vi "Bundler_Move Up Down Element Order.vi"(7 "Action":T2=enum."Bundler Move Up", 10 "Cluster Elements In":T1[](array[typedef]), 11 "Affected Items":T3) -> (3 "Cluster Elements Out":T1[](array[typedef]))   [LabVIEW 2023]
uses:
  top/BundleMagic.ctl
  controls/action enum.ctl
  Cluster Element Description.ctl
panel:
  # "Using Bundler Move Up and Bundler Move Down only"
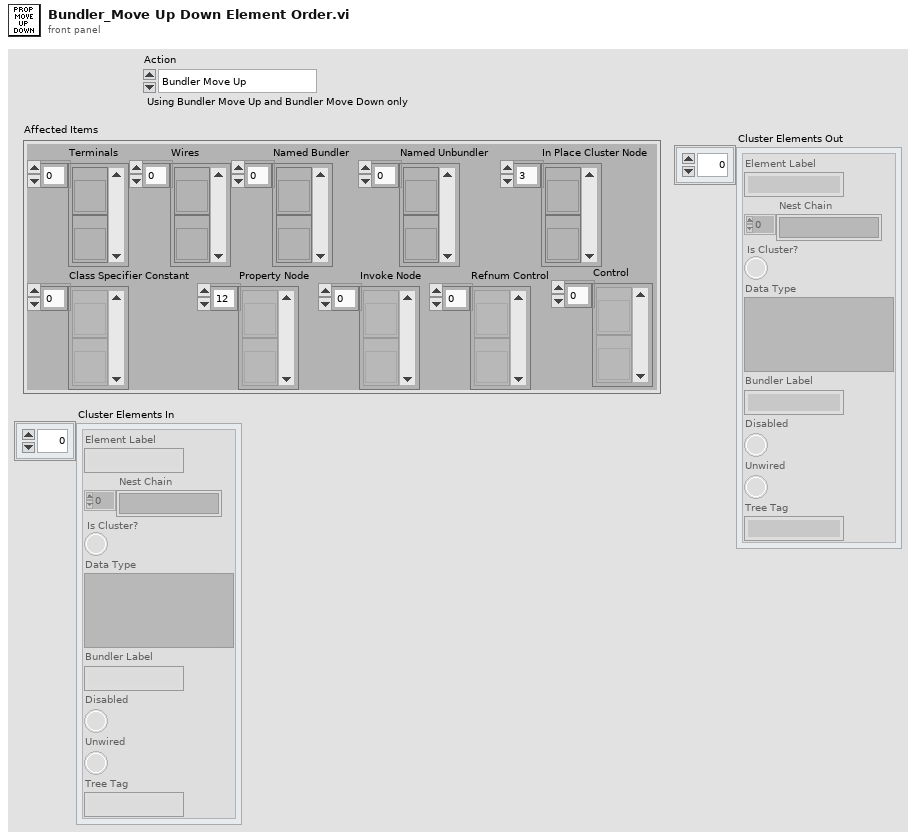
[diagram p1: front panel]
types:
  T1 = typedef "Cluster Element Description.ctl" = cluster{"Element Label":string, "Nest Chain":string[], "Is Cluster?":bool, "Data Type":variant, "Bundler Label":string, "Disabled":bool, "Unwired":bool, "Tree Tag":string}
  T2 = typedef "action enum.ctl" = enum16{"[NONE]", "Wire Bundle", "Wire Unbundle", "Terminal Unbundle", "Terminal Bundle", "Bundler Move Up", "Bundler Move Down", "Bundler Insert", "Bundler Remove", "Bundler Remove Unwired", "Bundler Rearrange", "In Place Insert", "In Place Remove", "In Place Remove Unwired", "In Place Rearrange", "Wire Properties", "Wire Method", "Terminal Properties", "Terminal Method", "Property Move Up", "Property Move Down", "Properties Insert", "Properties Remove", "Properties Remove Unwired", "Properties Rearrange", "Method Change", "Class for Constant", "Class For Control", "Class For Node", "Class Name to Clipboard"}
  T3 = typedef "BundleMagic.ctl" = cluster{"Terminals":refnum<vi>[], "Wires":refnum<vi>[], "Named Bundler":refnum<vi>[], "Named Unbundler":refnum<vi>[], "In Place Cluster Node":refnum<vi>[], "Class Specifier Constant":refnum<vi>[], "Property Node":refnum<vi>[], "Invoke Node":refnum<vi>[], "Refnum Control":refnum<vi>[], "Control":refnum<vi>[]}
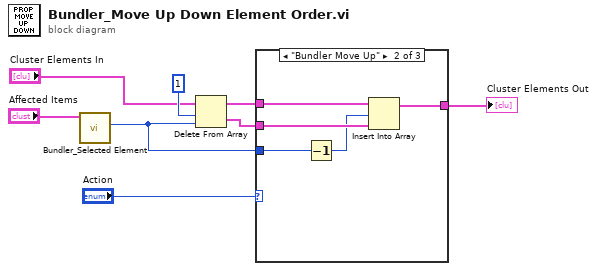
[diagram p0: block diagram]
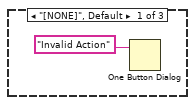
[diagram p2: hidden frame]
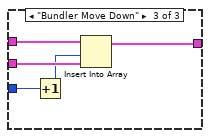
[diagram p3: hidden frame]
diagram:
  n1 = call "Bundler_Selected Element.vi"("Affected Items"="Affected Items") -> ("index of element"=w2:i32)  [unwired: 5 in, 5 out]
  n2 = Delete From Array(array="Cluster Elements In", length=1 ("index of element"), index=w2) -> (deleted portion=w6:T1[], array with subset deleted=w7:T1[])
  n3 = case shown="\"Bundler Move Up\"" "Action" {
    tunnel: w7 -> [_ w14 w19]
    tunnel: w6 -> [_ w13 w18]
    tunnel: w2 -> [_ w12 w16]
    tunnel: [_ w10 w17] -> w4
    frame "[NONE]", Default {
      n4 = One Button Dialog(message="Invalid Action") -> ()  [unwired: 1 in, 1 out]
    }
    frame "Bundler Move Up" {
      n5 = Decrement(x=w12) -> (x-1=w11:i32)
      n6 = Insert Into Array(array=w14, index=w11, new element=w13) -> (w10:T1[])
    }
    frame "Bundler Move Down" {
      n7 = Increment(x=w16) -> (x+1=w15:i32)
      n8 = Insert Into Array(array=w19, index=w15, new element=w18) -> (w17:T1[])
    }
  }
  "Cluster Elements Out" <- w4
